vi "VNARP-CASES.vi"(5 "entrée d'erreur (pas d'erreur)":errorcluster, 6 "Setting":u32=400000, 7 "Énum":T1(ring), 8 "ID de connexion":refnum<k5>) -> (0 "sortie d'erreur":errorcluster, 3 "ID de connexion en sortie":refnum<k5>)   [LabVIEW 2021]
panel:
  out "entier 32 bits non signé":u32
  out "x << y":u32
  out "entier 16 bits":i16
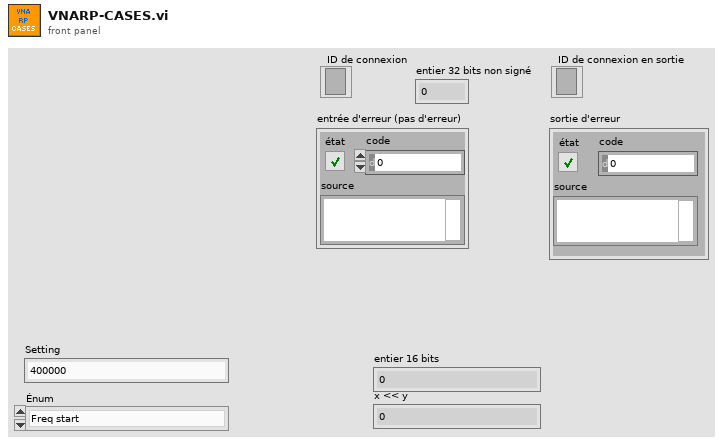
[diagram p1: front panel]
types:
  T1 = enum16{"Freq start", "Freq stop", "Sweep size", "Decimation rate", "Freq corr", "Phase output 1", "Phase output 2", "Output level 1", "Output level 2", "GPIO", "SWEEP START"}
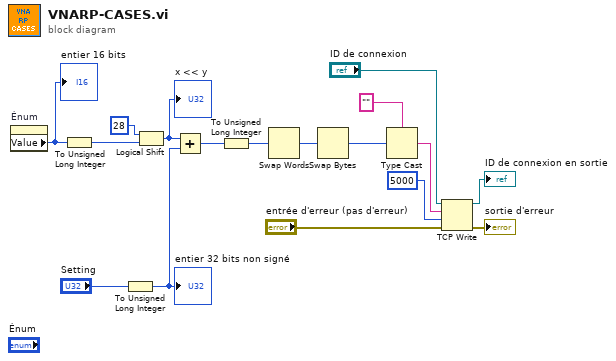
[diagram p0: block diagram]
diagram:
  n1 = property on="Énum" class="Enum (strict)"() -> ("Value"=w1:T1)  [unwired: 2 in, 2 out]
  "entier 16 bits" <- w1
  n2 = To Unsigned Long Integer(number=w1) -> (unsigned 32bit integer=w2:u32)
  n3 = To Unsigned Long Integer(number="Setting") -> (unsigned 32bit integer=w17:u32)
  "entier 32 bits non signé" <- w17
  n4 = Logical Shift(y=i16 28 ("n"), x=w2) -> (x << y=w14:u32)
  "x << y" <- w14
  n5 = Add(x=w14, y=w17) -> (x+y=w16:u32)
  n6 = To Unsigned Long Integer(number=w16) -> (unsigned 32bit integer=w9:u32)
  n7 = Swap Words(1:w9) -> (0:w10:u32)
  n8 = Swap Bytes(anything=w10) -> (byte swapped=w11:u32)
  n9 = Type Cast(type="", x=w11) -> (*(type *) &x=w12:string)
  n10 = TCP Write(connection ID="ID de connexion", data in=w12, error in (no error)="entrée d'erreur (pas d'erreur)", 9:5000 ("timeout en ms (25000)")) -> (connection ID out=→"ID de connexion en sortie":refnum<k5>, error out=→"sortie d'erreur":errorcluster)  [unwired: 1 out]
